vi "Transform Lidar Data to Cartesian Grid.vi"(10 "Bot Angle (rad)":dbl, 11 "Lidar Data (mm, rad)":cluster{dbl[], dbl[]}) -> (3 "Cartesian Lidar Data":cluster{"X":dbl, "Y":dbl}[](array[cluster]))   [LabVIEW 2017]
panel:
  out "XY Graph":cluster{"X":dbl, "Y":dbl}[](graph)
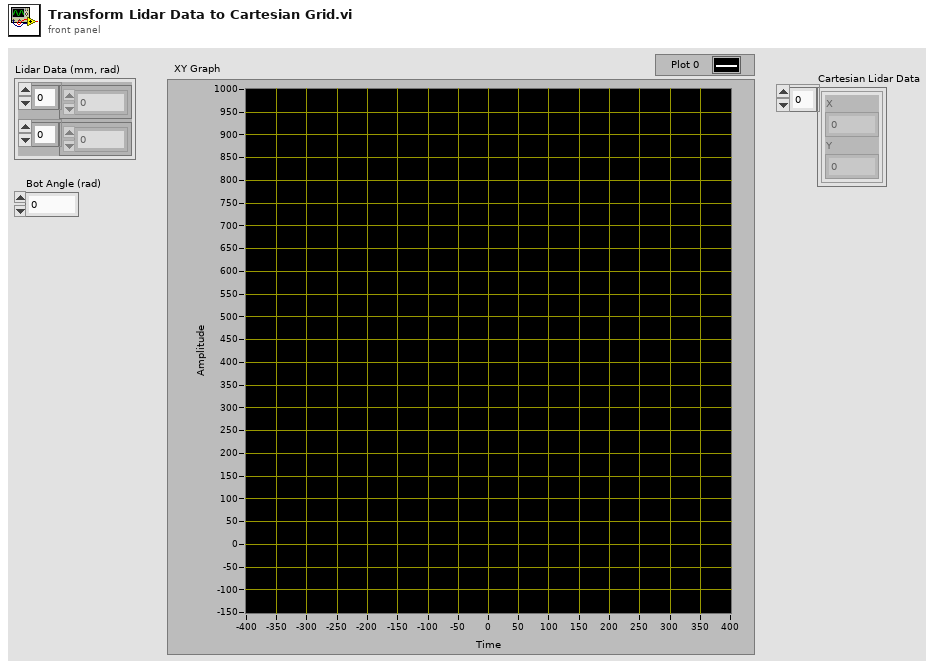
[diagram p1: front panel]
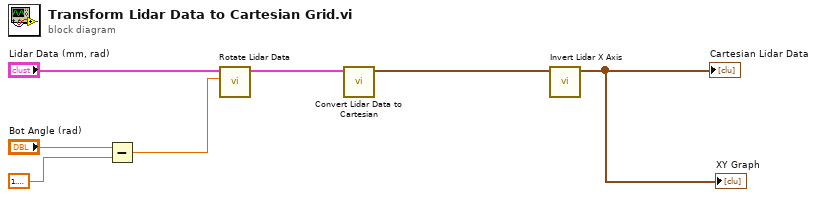
[diagram p0: block diagram]
diagram:
  n1 = Subtract(x="Bot Angle (rad)", y=1.5707963267948966) -> (x-y=w3:dbl)
  n2 = call "Rotate Lidar Data.vi"("Angle (rad)"=w3, "Raw Lidar Data"="Lidar Data (mm, rad)") -> ("Rotated Lidar Data"=w7:cluster{dbl[], dbl[]})  [unwired: 9 in]
  n3 = call "Convert Lidar Data to Cartesian.vi"("Polar Lidar Data"=w7) -> ("Cartesian Lidar Data"=w2:cluster{"X":dbl, "Y":dbl}[])  [unwired: 10 in]
  n4 = call "Invert Lidar X Axis.vi"("Cartesian Lidar Data"=w2) -> ("Inverted Lidar Data"=→"Cartesian Lidar Data" →"XY Graph":cluster{"X":dbl, "Y":dbl}[])  [unwired: 10 in]
